vi "getDeviceStatus.vi"(8 "error in (no error)":errorcluster, 11 "tcpDevice in":refnum<class "tcpDevice.lvclass">) -> (0 "error out":errorcluster, 2 "status":T1, 3 "tcpDevice out":refnum<class "tcpDevice.lvclass">)   [LabVIEW 2016, in "tcpDevice.lvclass"]
uses:
  tcpDevice.lvclass
  typedefs/deviceStatus.ctl
  typedefs/statusEnum.ctl
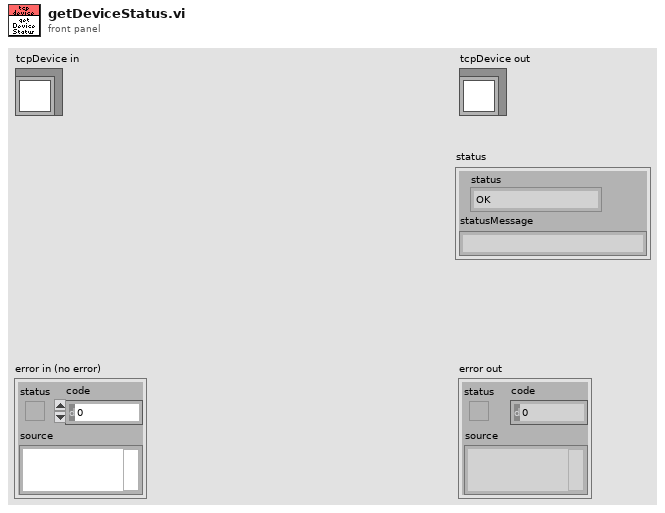
[diagram p1: front panel]
types:
  T1 = typedef "deviceStatus.ctl" = cluster{"status":T2, "statusMessage":string}
  T2 = typedef "statusEnum.ctl" = enum16{"OK", "TIMEOUT", "MSGERROR"}
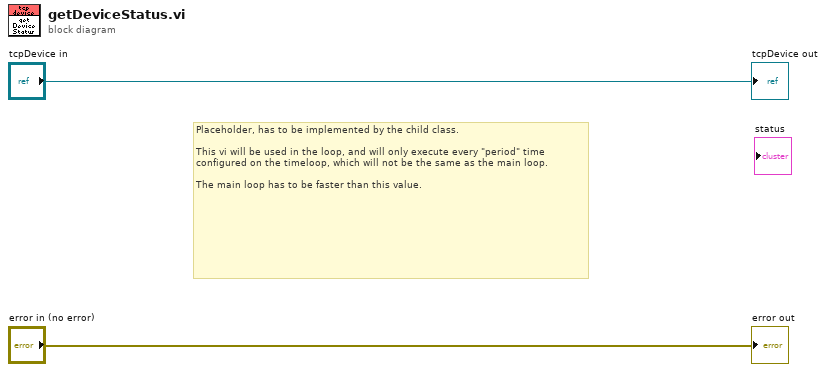
[diagram p0: block diagram]
diagram:
  # "Placeholder, has to be implemented by the child class.\n\nThis vi will be used in the loop, and will only execute every \"period\" time configured on the timeloop, which will not be the same as the main loop.\n\nThe main loop has to be faster than this value."
  "error out" <- "error in (no error)"
  "tcpDevice out" <- "tcpDevice in"
